vi "doAction.vi"(8 "error in (no error)":errorcluster, 10 "ContextData":refnum<class "ContextData.lvclass">, 11 "User State 2 in":refnum<class "User State 2.lvclass">) -> (0 "error out":errorcluster, 2 "ContextData Out":refnum<class "ContextData.lvclass">, 3 "User State 2 out":refnum<class "User State 2.lvclass">)   [LabVIEW 2019, in "User State 2.lvclass"]
uses:
  User State 2.lvclass
  ContextData/ContextData.lvclass
  ContextData/ContextData.lvclass/ContextData.ctl
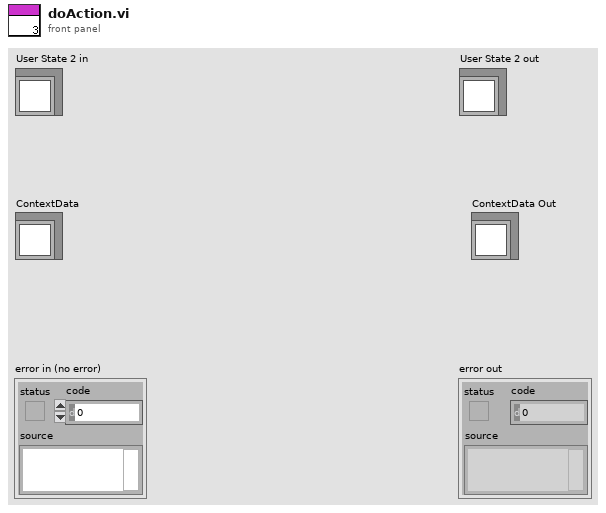
[diagram p1: front panel]
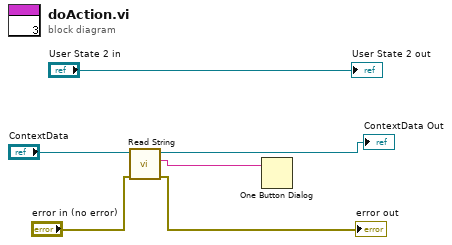
[diagram p0: block diagram]
diagram:
  n1 = call "Read String.vi"("error in (no error)"="error in (no error)", "ContextData in"="ContextData") -> ("error out"=→"error out":errorcluster, "String <Replace Me>"=w4:string, "ContextData out"=→"ContextData Out":refnum<class "ContextData.lvclass">)  [unwired: 7 in]
  n2 = One Button Dialog(message=w4) -> ()  [unwired: 1 in, 1 out]
  "User State 2 out" <- "User State 2 in"
